vi "SaveWaveformDataDVR.vi"(6 "Registry":T17, 7 "data event data":T3, 8 "error in (no error)":errorcluster, 9 "dataflow type":T2, 10 "Waveforms":T1, 11 "data event":T11) -> (0 "error out":errorcluster, 3 "data event data out":T3)   [LabVIEW 2017, in "CmsDataEventCreator.lvlib"]
uses:
  <vilib>/addons/InsightCM/Devices/Shared/Cms/CmsDataEventCreator/CmsDataEventCreator.lvlib
  <vilib>/addons/InsightCM/Devices/Shared/Cms/CmsDataEventCreator/controls/GroupRegistry.ctl
  <vilib>/addons/InsightCM/Devices/Shared/Cms/CmsDataEventCreator/controls/DataSetRegistry.ctl
  <vilib>/addons/InsightCM/Devices/Shared/Common/DataEvent/controls/DataSetType.ctl
  <vilib>/addons/InsightCM/Devices/Shared/Common/DataEventCreator/controls/Registry_Trend.ctl
  <vilib>/addons/InsightCM/Devices/Shared/Cms/CmsDataEventCreator/controls/DataEventConfig.ctl
  <vilib>/addons/InsightCM/Devices/Shared/Cms/CmsDataEventCreator/controls/AcqParams.ctl
  <vilib>/addons/InsightCM/Devices/Shared/Common/DataAccumulator/controls/AccumulationSettings.ctl
  <vilib>/addons/InsightCM/Devices/Shared/Common/DataAccumulator/controls/accumulationType.ctl
  <vilib>/addons/InsightCM/Devices/Shared/Common/DVRBuffer/controls/BufferLocation.ctl
  <vilib>/addons/PointValueMap/controls/PointMap.ctl
  <vilib>/addons/InsightCM/Devices/Shared/Common/DataEvent/controls/Event.ctl
  <vilib>/addons/InsightCM/MessageBus/Base/controls/DataEvent.ctl
  <vilib>/addons/InsightCM/MessageBus/Base/controls/KeyValuePair.ctl
  <vilib>/addons/InsightCM/Devices/Shared/Common/DataEvent/controls/DataSet.ctl
  <vilib>/addons/InsightCM/MessageBus/Base/controls/DataSetMetadata.ctl
  <vilib>/addons/InsightCM/MessageBus/Base/controls/TrendPoint.ctl
  <vilib>/addons/InsightCM/MessageBus/Base/controls/TrendAlarmUpdate.ctl
  <vilib>/addons/InsightCM/MessageBus/Base/controls/TrendAlarmTransition.ctl
  <vilib>/addons/InsightCM/Devices/Shared/Common/DataFlow/controls/Type.ctl
  <vilib>/addons/InsightCM/Utilities/DataAccessors/controls/wfmSGL_DVR.ctl
  <vilib>/addons/InsightCM/Devices/Shared/Common/DataFlow/DataFlow.lvlib
  <vilib>/addons/PointValueMap/PointValueMap.lvlib
  <vilib>/addons/InsightCM/Devices/Shared/Common/DataEvent/DataEvent.lvlib
  <vilib>/addons/InsightCM/Devices/Shared/Common/DataEventCreator/DataEventCreator.lvlib
  <vilib>/addons/InsightCM/Devices/Shared/Common/DataAccumulator/DataAccumulator.lvlib
  <vilib>/addons/InsightCM/Devices/Shared/Common/DVRBuffer/DVRBuffer.lvlib
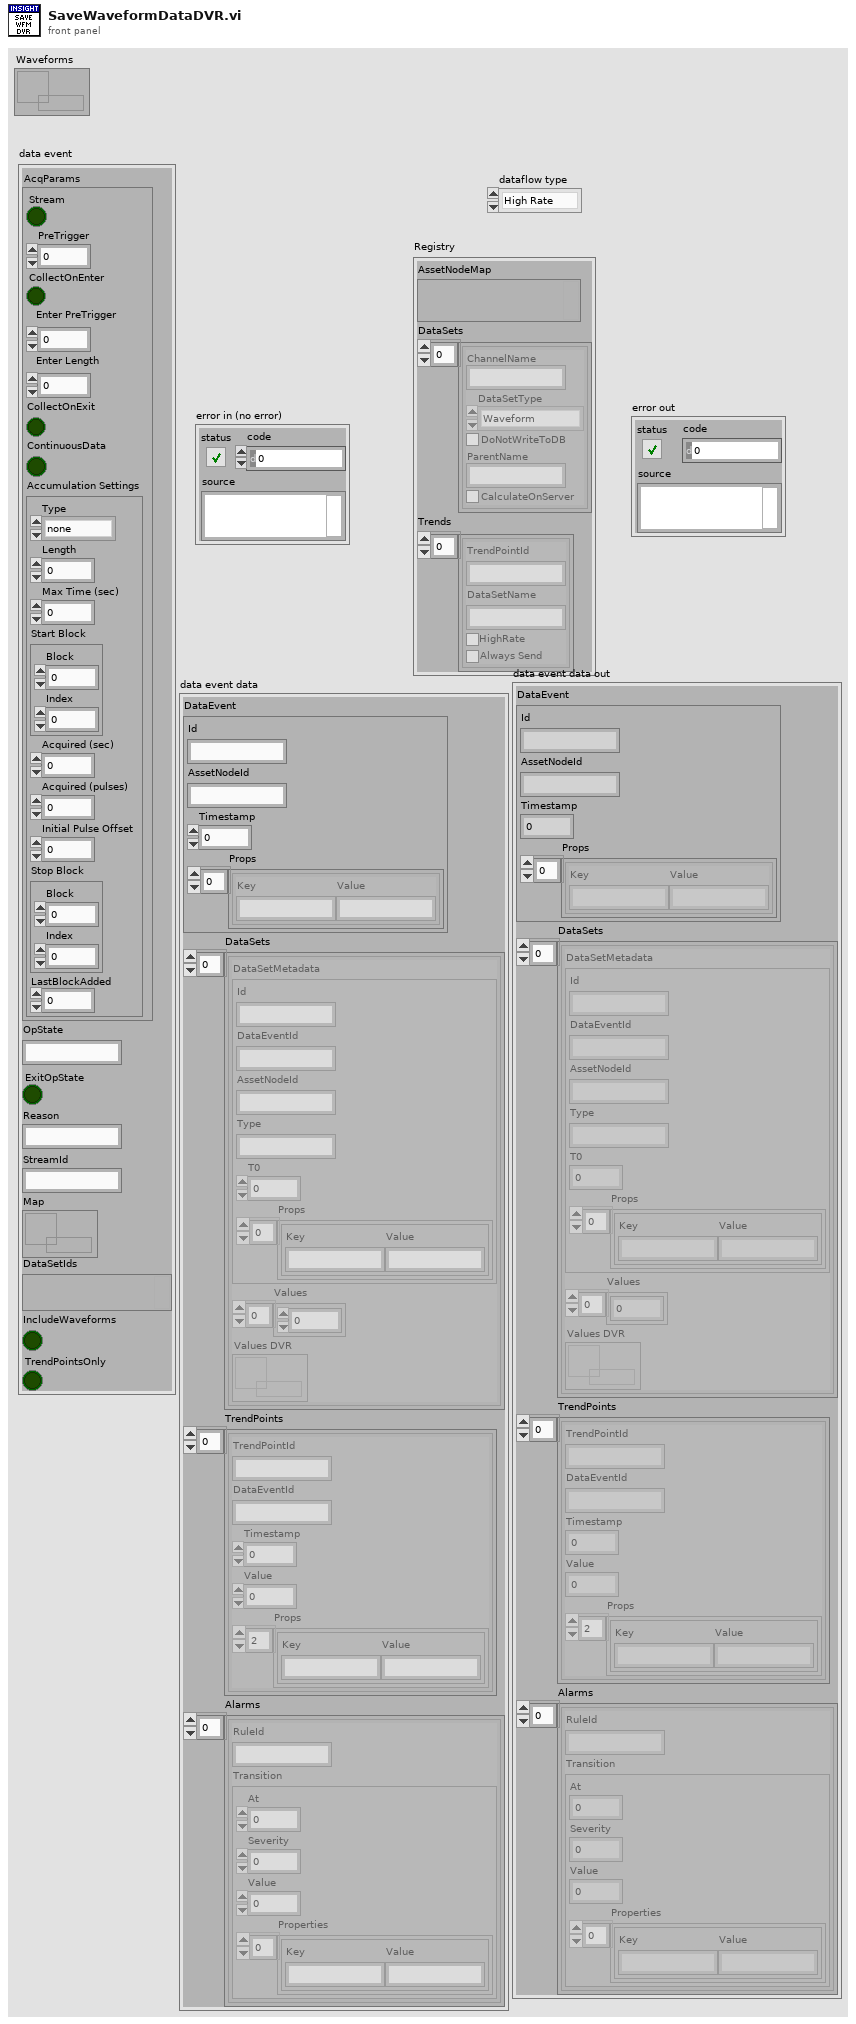
[diagram p1: front panel]
types:
  T1 = typedef "wfmSGL_DVR.ctl" = refnum<data-value>
  T2 = typedef "DataFlow.lvlib/Type.ctl" = enum16{"High Rate", "Low Rate", "Burst Mode"}
  T3 = typedef "DataEvent.lvlib/Event.ctl" = cluster{"DataEvent":T4, "DataSets":T6[], "TrendPoints":T8[], "Alarms":T9[]}
  T4 = typedef "DataEvent.ctl" = cluster{"Id":string, "AssetNodeId":string, "Timestamp":i64, "Props":T5[]}
  T5 = typedef "KeyValuePair.ctl" = cluster{"Key":string, "Value":string}
  T6 = typedef "DataEvent.lvlib/DataSet.ctl" = cluster{"DataSetMetadata":T7, "Values":sgl[], "Values DVR":refnum<data-value>}
  T7 = typedef "DataSetMetadata.ctl" = cluster{"Id":string, "DataEventId":string, "AssetNodeId":string, "Type":string, "T0":i64, "Props":T5[]}
  T8 = typedef "TrendPoint.ctl" = cluster{"TrendPointId":string, "DataEventId":string, "Timestamp":i64, "Value":dbl, "Props":T5[]}
  T9 = typedef "TrendAlarmUpdate.ctl" = cluster{"RuleId":string, "Transition":T10}
  T10 = typedef "TrendAlarmTransition.ctl" = cluster{"At":i64, "Severity":i32, "Value":dbl, "Properties":T5[]}
  T11 = typedef "CmsDataEventCreator.lvlib/DataEventConfig.ctl" = cluster{"AcqParams":T12, "OpState":string, "ExitOpState":bool, "Reason":string, "StreamId":string, "Map":T16, "DataSetIds":variant, "IncludeWaveforms":bool, "TrendPointsOnly":bool}
  T12 = typedef "CmsDataEventCreator.lvlib/AcqParams.ctl" = cluster{"Stream":bool, "PreTrigger":i32, "CollectOnEnter":bool, "Enter PreTrigger":i32, "Enter Length":dbl, "CollectOnExit":bool, "ContinuousData":bool, "Accumulation Settings":T13}
  T13 = typedef "DataAccumulator.lvlib/AccumulationSettings.ctl" = cluster{"Type":T14, "Length":dbl, "Max Time (sec)":dbl, "Start Block":T15, "Acquired (sec)":dbl, "Acquired (pulses)":i32, "Initial Pulse Offset":dbl, "Stop Block":T15, "LastBlockAdded":u32}
  T14 = typedef "DataAccumulator.lvlib/accumulationType.ctl" = enum16{"none", "seconds", "revolutions"}
  T15 = typedef "DVRBuffer.lvlib/BufferLocation.ctl" = cluster{"Block":u32, "Index":i32}
  T16 = typedef "PointValueMap.lvlib/PointMap.ctl" = refnum<data-value>
  T17 = typedef "CmsDataEventCreator.lvlib/GroupRegistry.ctl" = cluster{"AssetNodeMap":variant, "DataSets":T18[], "Trends":T20[]}
  T18 = typedef "CmsDataEventCreator.lvlib/DataSetRegistry.ctl" = cluster{"ChannelName":string, "DataSetType":T19, "DoNotWriteToDB":bool, "ParentName":string, "CalculateOnServer":bool}
  T19 = typedef "DataEvent.lvlib/DataSetType.ctl" = enum16{"Waveform", "SpeedProfile", "ThermalImage", "EmsaSweep"}
  T20 = typedef "DataEventCreator.lvlib/Registry_Trend.ctl" = cluster{"TrendPointId":string, "DataSetName":string, "HighRate":bool, "Always Send":bool}
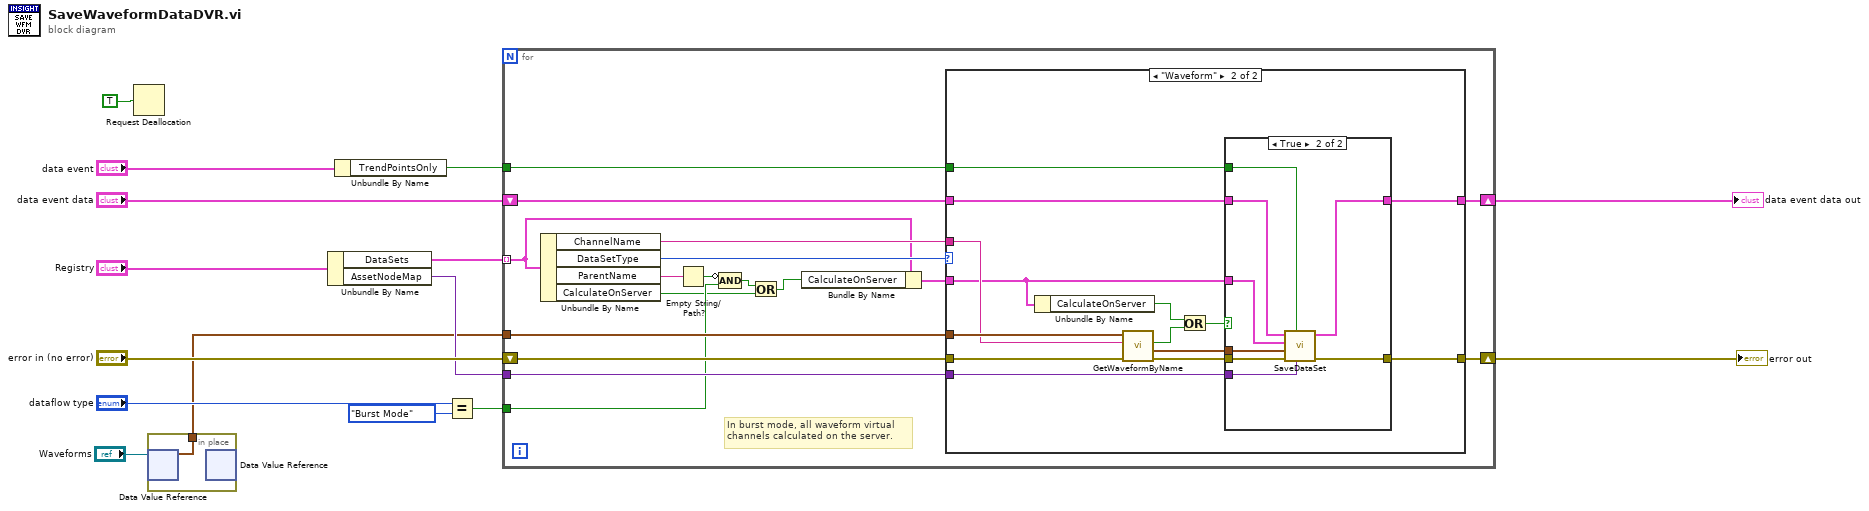
[diagram p0: block diagram]
diagram:
  n1 = Request Deallocation(TRUE ("flag")) -> ()
  n2 = in-place {
    in-place-border: [w16] -> w1
    n3 = in-place-dvr #1("Waveforms") -> (w16:waveform(sgl)[])  [unwired: 1 out]
    n4 = in-place-dvr #1() -> ()  [unwired: 1 in, 2 out]
  }
  n5 = Unbundle By Name("Registry") -> ("DataSets"=w13:T18[], "AssetNodeMap"=w11:variant)
  n6 = Unbundle By Name("data event") -> ("TrendPointsOnly"=w10:bool)
  n7 = Equal?(x="dataflow type", y=Type."Burst Mode") -> (x = y?=w3:bool)
  n8 = for {
    tunnel: w1 -> [w32]
    tunnel: w13 -> [w24] mode=indexing
    shift-right: [w31] -> w12
    shift-left: "error in (no error)" -> [w33]
    tunnel: w11 -> [w27]
    shift-right: [w26] -> w7
    shift-left: "data event data" -> [w28]
    tunnel: w10 -> [w25]
    tunnel: w3 -> [w22]
    # "In burst mode, all waveform virtual\nchannels calculated on the server."
    n9 = Unbundle By Name(w24) -> ("ChannelName"=w30:string, "DataSetType"=w29:T19, "ParentName"=w20:string, "CalculateOnServer"=w18:bool)
    n10 = Empty String/Path?(string/path=w20) -> (empty?=w21:bool)
    n11 = Compound Arithmetic op=AND(invert w21, w22) -> (w19:bool)
    n12 = Or(x=w19, y=w18) -> (x .or. y?=w17:bool)
    n13 = Bundle By Name(cluster=w24, "CalculateOnServer"=w17) -> (w23:T18)
    n14 = case shown="\"Waveform\"" w29 {
      tunnel: w33 -> [w34 w40]
      tunnel: w32 -> [_ w49]
      tunnel: [w34 w48] -> w31
      tunnel: w30 -> [_ w47]
      tunnel: w28 -> [w35 w46]
      tunnel: w27 -> [_ w45]
      tunnel: w23 -> [_ w39]
      tunnel: [w35 w44] -> w26
      tunnel: w25 -> [_ w43]
      frame Default {
      }
      frame "Waveform" {
        n15 = Unbundle By Name(w39) -> ("CalculateOnServer"=w38:bool)
        n16 = call <vilib>:"GetWaveformByName.vi"("error in (no error)"=w40, "Channel Name"=w47, "Acq Waveforms"=w49) -> ("error out"=w42:errorcluster, "Waveform"=w41:waveform(sgl), "Found?"=w37:bool)  [unwired: 5 in, 1 out]
        n17 = Or(x=w38, y=w37) -> (x .or. y?=w36:bool)
        n18 = case shown="True" w36 {
          tunnel: w42 -> [w51 w59]
          tunnel: w41 -> [_ w58]
          tunnel: [w51 w53] -> w48
          tunnel: w46 -> [w50 w57]
          tunnel: w45 -> [_ w56]
          tunnel: w39 -> [_ w55]
          tunnel: [w50 w54] -> w44
          tunnel: w43 -> [_ w52]
          frame False {
          }
          frame True {
            n19 = call <vilib>:"SaveDataSet.vi"("AssetNodeMap"=w56, "do not write to database"=w52, "error in (no error)"=w59, "Waveform"=w58, "DataSetRegistry"=w55, "event in"=w57) -> ("error out"=w53:errorcluster, "event out"=w54:T3)  [unwired: 4 in]
          }
        }
      }
    }
  }
  "error out" <- w12
  "data event data out" <- w7
